vi "DiagramFactory.vi"(8 "error in":errorcluster, 11 "reference":refnum<vi>) -> (0 "error out":errorcluster, 3 "Diagram out":refnum<class "Diagram.lvclass">)   [LabVIEW 2014, in "Diagram.lvclass"]
uses:
  Diagram.lvclass
  TopLevelDiagram/TopLevelDiagram.lvclass
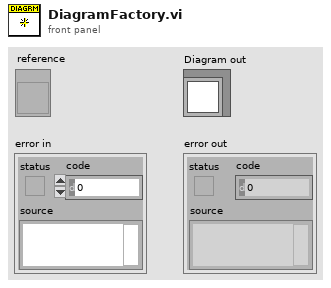
[diagram p1: front panel]
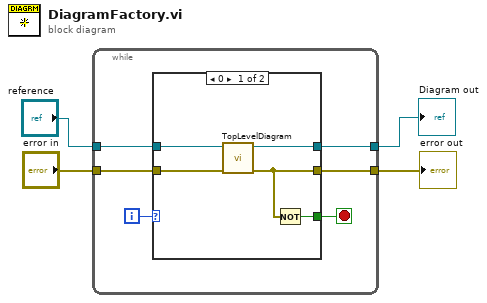
[diagram p0: block diagram]
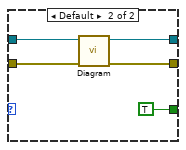
[diagram p2: hidden frame]
diagram:
  n1 = while {
    tunnel: "reference" -> [w9]
    tunnel: "error in" -> [w8]
    tunnel: [w7] -> w1
    tunnel: [w6] -> w2
    i -> [w10]
    stop <- w5 stop-if-true
    n2 = case shown="0" w10 {
      tunnel: w9 -> [w14 w18]
      tunnel: w8 -> [w15 w19]
      tunnel: [w11 w17] -> w7
      tunnel: [w13 w20] -> w6
      tunnel: [w12 TRUE] -> w5
      frame 0 {
        n3 = call "TopLevelDiagram.vi"("error in"=w15, "reference"=w14) -> ("error out"=w11:errorcluster, "TopLevelDiagram out"=w13:refnum<class "TopLevelDiagram.lvclass">)  [unwired: 8 in]
        n4 = Not(x=w11) -> (.not. x?=w12:bool)
      }
      frame Default {
        n5 = call "Diagram.vi"("error in"=w19, "reference"=w18) -> ("error out"=w17:errorcluster, "Diagram out"=w20:refnum<class "Diagram.lvclass">)  [unwired: 8 in]
      }
    }
  }
  "error out" <- w1
  "Diagram out" <- w2
